vi "断电保存变量.vi"() -> ()   [LabVIEW 2016, in "PLC.lvlib"]
uses:
  PLC.lvlib
panel:
  in  "AD线性关系":T1(array[cluster])=[{"X0"=1638.0, "X1"=8191.0, "Y0"=-40.0, "Y1"=100.0}, {"X0"=1638.0, "X1"=8191.0, "Y0"=0.0, "Y1"=100.0}, {"X0"=1638.0, "X1"=8191.0, "Y0"=0.0, "Y1"=1.0}, {"X0"=0.0, "X1"=8191.0, "Y0"=0.0, "Y1"=8191.0}, {"X0"=0.0, "X1"=8191.0, "Y0"=0.0, "Y1"=8191.0}, {"X0"=0.0, "X1"=8191.0, "Y0"=0.0, "Y1"=8191.0}]
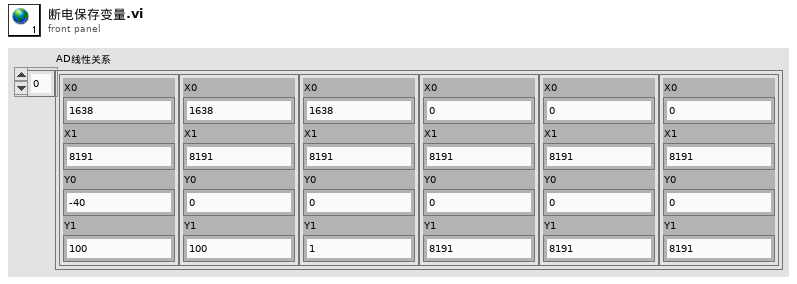
[diagram p1: front panel]
types:
  T1 = cluster{"X0":dbl, "X1":dbl, "Y0":dbl, "Y1":dbl}[]
diagram:
